vi "damped sinusoid fit BAP2B.vi"(7 "fitting parameters":T1 {"decay rate (1/sec)" scale=0.0..20000.0; "start phase (deg)" scale=-180.0..180.0; "frequency (Hz)" scale=0.0..20000.0; "amplitude (V)" scale=0.0..10.0}, 11 "time array in (s)":dbl[](array[numeric])) -> (0 "parameters array out":dbl[](array[numeric]), 2 "voltage array out (V)":dbl[](array[numeric]), 3 "time array out (s)":dbl[](array[numeric]))   [LabVIEW 2014]
doc: "damped sinusoid fit BAP2B\n\nTakes an array of times [s], along with fitting parameters (amplitude[V], angular frequency[1/s], phase shift [rad] and decay rate [1/s]) to produce an array of voltages , return the time array, and convert the cluster of parameters into another array.\n\nCalculations:\nv(t) = A^(-gt) * sint(wt +p)\n\nBeverly Abadines\nPhy 350\nBAP2B"
uses:
  typedefs/damped wave parameter cluster.ctl
panel:
  # "Beverly Abadines\nPHY 350\nBAP2B"
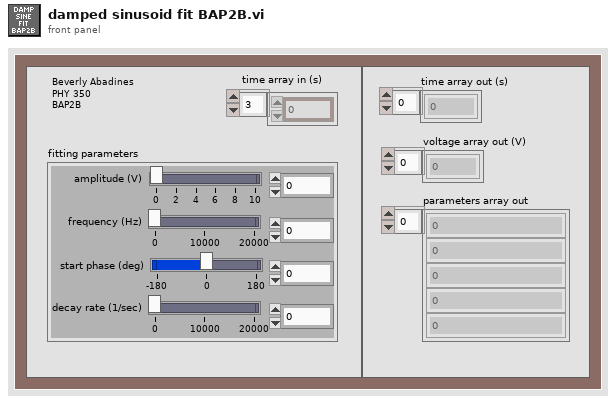
[diagram p1: front panel]
types:
  T1 = typedef "damped wave parameter cluster.ctl" = cluster{"amplitude (V)":dbl, "frequency (Hz)":dbl, "start phase (deg)":dbl, "decay rate (1/sec)":dbl}
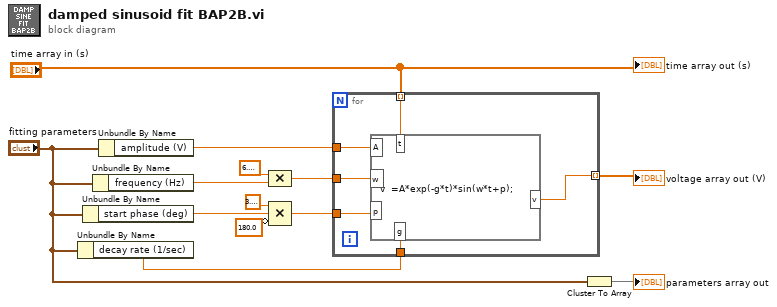
[diagram p0: block diagram]
diagram:
  n1 = Unbundle By Name("fitting parameters") -> ("decay rate (1/sec)"=w4:dbl)
  n2 = Unbundle By Name("fitting parameters") -> ("start phase (deg)"=w9:dbl)
  n3 = Unbundle By Name("fitting parameters") -> ("frequency (Hz)"=w10:dbl)
  n4 = Unbundle By Name("fitting parameters") -> ("amplitude (V)"=w8:dbl)
  n5 = Compound Arithmetic op=MULTIPLY(6.283185307179586, w10) -> (w5:dbl)
  n6 = Compound Arithmetic op=MULTIPLY(3.141592653589793, w9, invert 180.0 ("value")) -> (w6:dbl)
  n7 = for {
    tunnel: w8 -> [w19]
    tunnel: "time array in (s)" -> [w14] mode=indexing
    tunnel: w6 -> [w18]
    tunnel: w5 -> [w17]
    tunnel: w4 -> [w16]
    tunnel: [w15] -> w1 mode=indexing
    n8 = formula code="v  =A*exp(-g*t)*sin(w*t+p);"("A"=w19, "t"=w14, "w"=w17, "p"=w18, "g"=w16) -> ("v"=w15:dbl)
  }
  "voltage array out (V)" <- w1
  n9 = Cluster To Array(cluster="fitting parameters") -> (array=→"parameters array out":dbl[])
  "time array out (s)" <- "time array in (s)"
